vi "Joystick State to XBox One Controller.vi"(10 "Joystick State":cluster{"Buttons":T3[], "Axis":T4[]}) -> (2 "Xbox One Controller":T1 {"Right Joystick"."Right" min=-1.0 max=1.0 step=0.1 scale=-1.0..1.0; "Right Joystick"."Forward" min=-1.0 max=1.0 step=0.1 scale=-1.0..1.0; "Left Joystick"."Right" min=-1.0 max=1.0 step=0.1 scale=-1.0..1.0; "Left Joystick"."Forward" min=-1.0 max=1.0 step=0.1 scale=-1.0..1.0})   [LabVIEW 2014, in "Xbox One Controller.lvlib"]
uses:
  Xbox One Controller.lvlib
  Joystick/Joystick Class/Button State.ctl
  Joystick/Joystick Class/Axis State.ctl
  Xbox One Controller State.ctl
  Joystick.ctl
  Joystick/Joystick Class/Joystick.lvclass
panel:
  in  "Stateful Only":bool
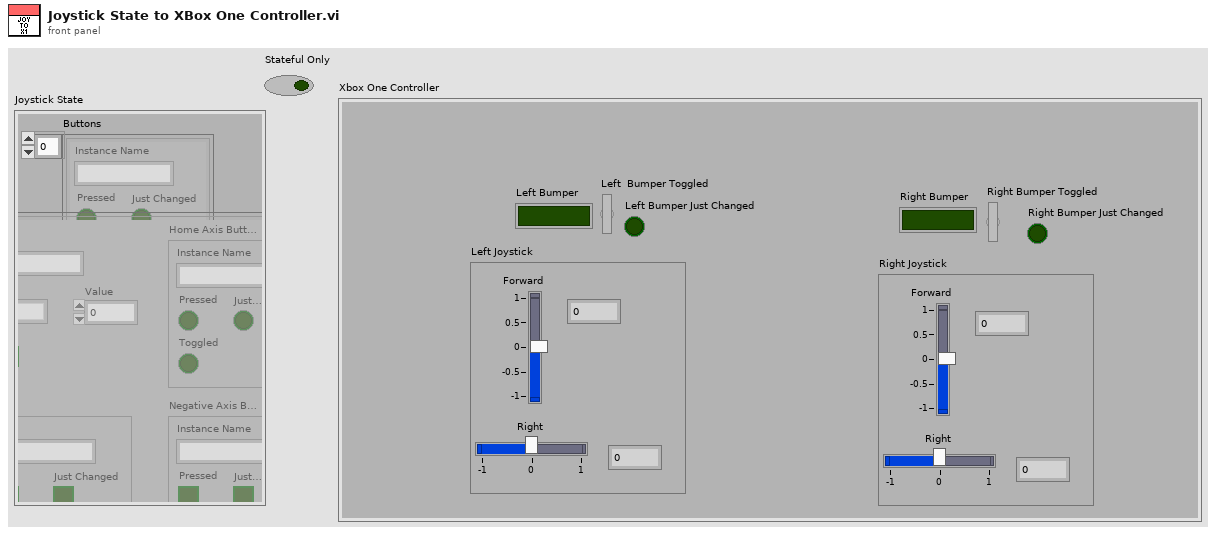
[diagram p1: front panel]
types:
  T1 = typedef "Xbox One Controller.lvlib/Xbox One Controller State.ctl" = cluster{"Left Joystick":T2, "Right Joystick":T2, "Right Bumper":bool, "Left Bumper":bool, "Left  Bumper Toggled":bool, "Right Bumper Toggled":bool, "Left Bumper Just Changed":bool, "Right Bumper Just Changed":bool}
  T2 = typedef "Xbox One Controller.lvlib/Joystick.ctl" = cluster{"Forward":dbl, "Right":dbl}
  T3 = typedef "Joystick.lvlib/Joystick.lvclass/Button State.ctl" = cluster{"Pressed":bool, "Instance Name":string, "Toggled":bool, "Just Changed":bool}
  T4 = typedef "Joystick.lvlib/Joystick.lvclass/Axis State.ctl" = cluster{"Instance Name":string, "Deadband":dbl, "Value":dbl, "At Home":bool, "Postive Axis Button State":T3, "Negative Axis Button State":T3, "Home Axis Button State":T3}
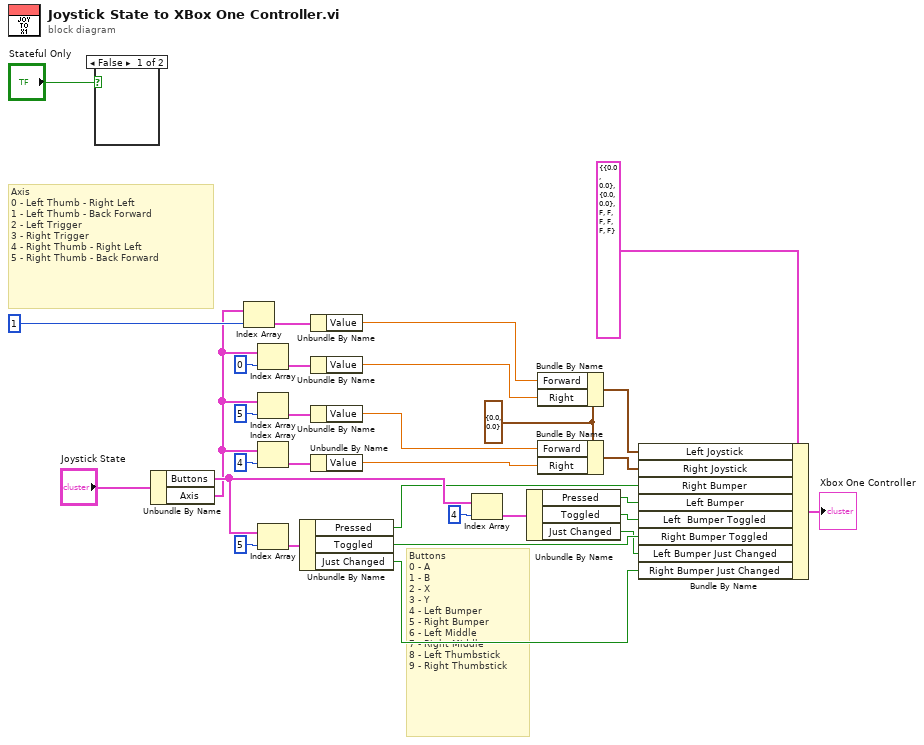
[diagram p0: block diagram]
diagram:
  w14 = T2 {"Forward"=0.0, "Right"=0.0} ("Left Joystick")
  # "Buttons\n0 - A\n1 - B\n2 - X\n3 - Y\n4 - Left Bumper\n5 - Right Bumper\n6 - Left Middle\n7 - Right Middle\n8 - Left Thumbstick\n9 - Right Thumbstick"
  # "Axis\n0 - Left Thumb - Right Left\n1 - Left Thumb - Back Forward\n2 - Left Trigger\n3 - Right Trigger\n4 - Right Thumb - Right Left\n5 - Right Thumb - Back Forward"
  n1 = case shown="False" "Stateful Only" {
    frame False {
    }
    frame True {
    }
  }
  n2 = Unbundle By Name("Joystick State") -> ("Buttons"=w23:T3[], "Axis"=w11:T4[])
  n3 = Index Array(array=w11, index=1) -> (element=w18:T4)
  n4 = Index Array(array=w11, index=0) -> (element=w19:T4)
  n5 = Index Array(array=w11, index=5) -> (element=w9:T4)
  n6 = Index Array(array=w11, index=4) -> (element=w10:T4)
  n7 = Index Array(array=w23, index=5) -> (element=w24:T3)
  n8 = Unbundle By Name(w24) -> ("Pressed"=w22:bool, "Toggled"=w4:bool, "Just Changed"=w2:bool)
  n9 = Unbundle By Name(w18) -> ("Value"=w16:dbl)
  n10 = Unbundle By Name(w19) -> ("Value"=w15:dbl)
  n11 = Unbundle By Name(w9) -> ("Value"=w7:dbl)
  n12 = Unbundle By Name(w10) -> ("Value"=w8:dbl)
  n13 = Index Array(array=w23, index=4) -> (element=w27:T3)
  n14 = Unbundle By Name(w27) -> ("Pressed"=w26:bool, "Toggled"=w5:bool, "Just Changed"=w3:bool)
  n15 = Bundle By Name(cluster=w14, "Forward"=w16, "Right"=w15) -> (w17:T2)
  n16 = Bundle By Name(cluster=w14, "Forward"=w7, "Right"=w8) -> (w6:T2)
  n17 = Bundle By Name(cluster=T1 {"Left Joystick"={"Forward"=0.0, "Right"=0.0}, "Right Joystick"={"Forward"=0.0, "Right"=0.0}, "Right Bumper"=FALSE, "Left Bumper"=FALSE, "Left  Bumper Toggled"=FALSE, "Right Bumper Toggled"=FALSE, "Left Bumper Just Changed"=FALSE, "Right Bumper Just Changed"=FALSE} ("Xbox One Controller"), "Left Joystick"=w17, "Right Joystick"=w6, "Right Bumper"=w22, "Left Bumper"=w26, "Left  Bumper Toggled"=w5, "Right Bumper Toggled"=w4, "Left Bumper Just Changed"=w3, "Right Bumper Just Changed"=w2) -> (→"Xbox One Controller":T1)
